vi "Clear Array.vi"(8 "error in (no error)":errorcluster, 11 "2DArrayManager in":refnum<class "2DArrayManager.lvclass">) -> (0 "error out":errorcluster, 3 "2DArrayManager out":refnum<class "2DArrayManager.lvclass">)   [LabVIEW 2020, in "OOPanel.lvlib" / "2DArrayManager.lvclass"]
doc: "Removes all panels from the layout but does NOT clean them up. They are marked as orphans so they can easily be reinserted as needed. Once orphaned, if the manager is cleaned up, the orphaned panels will be too."
uses:
  2DArrayManager.lvclass
  2DArrayManager.lvclass/2DArrayManager.ctl
  ArrayPanel/ArrayPanel.lvclass
  Panel/Panel.lvclass
  Manager/Manager.lvclass
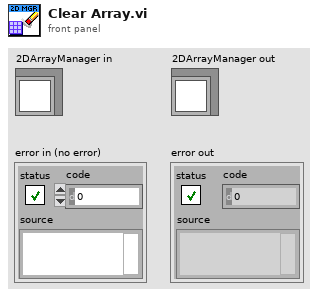
[diagram p1: front panel]
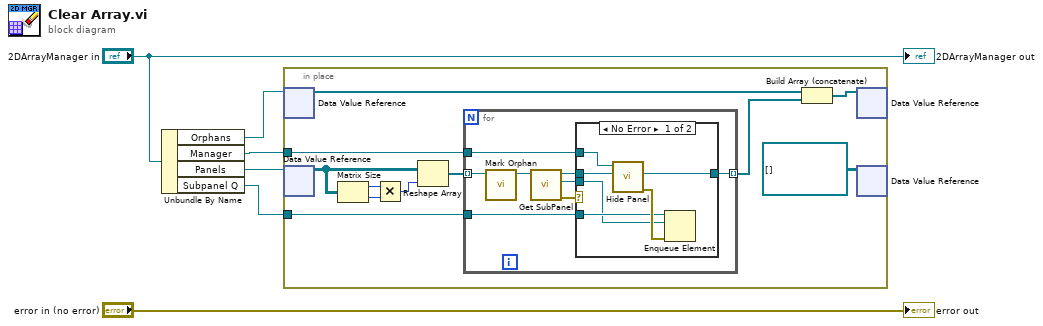
[diagram p0: block diagram]
diagram:
  n1 = Unbundle By Name("2DArrayManager in") -> ("Orphans"=w2:refnum<data-value>, "Manager"=w1:refnum<class "Manager.lvclass">, "Panels"=w4:refnum<data-value>, "Subpanel Q"=w3:refnum<queue>)
  n2 = in-place {
    in-place-border: w3 -> [w9]
    in-place-border: w1 -> [w8]
    n3 = in-place-dvr #1(w2) -> (w11:refnum<class "ArrayPanel.lvclass">[])  [unwired: 1 out]
    n4 = in-place-dvr #2(w4) -> (w17:refnum<class "ArrayPanel.lvclass">[][])  [unwired: 1 out]
    n5 = Matrix Size(0:w17) -> (1:w16:i32, 2:w15:i32)
    n6 = Multiply(x=w16, y=w15) -> (x*y=w14:i32)
    n7 = Reshape Array(w17, w14) -> (w12:refnum<class "ArrayPanel.lvclass">[])
    n8 = for {
      tunnel: w12 -> [w25] mode=indexing
      tunnel: w9 -> [w20]
      tunnel: w8 -> [w19]
      tunnel: [w18] -> w7 mode=indexing
      n9 = call "Mark Orphan.vi"("ArrayPanel in"=w25) -> ("ArrayPanel out"=w24:refnum<class "ArrayPanel.lvclass">)  [unwired: 9 in, 1 out]
      n10 = call "Get SubPanel.vi"("Panel in"=w24) -> ("error out"=w21:errorcluster, "SubPanel"=w22:refnum<vi>, "Panel out"=w23:refnum<class "ArrayPanel.lvclass">)  [unwired: 8 in]
      n11 = case shown="No Error" w21 {
        tunnel: w23 -> [w28 w32]
        tunnel: w22 -> [w27 _]
        tunnel: w20 -> [w30 _]
        tunnel: w19 -> [w29 _]
        tunnel: [w26 w32] -> w18
        frame No Error {
          n12 = call "Hide Panel.vi"("Panel In"=w28, "Manager in"=w29) -> ("error out"=w31:errorcluster, "Panel"=w26:refnum<class "ArrayPanel.lvclass">)  [unwired: 7 in, 1 out]
          n13 = Enqueue Element(queue=w30, element=w27, error in (no error)=w31) -> ()  [unwired: 1 in, 3 out]
        }
        frame Error {
        }
      }
    }
    n14 = Build Array (concatenate)(w11, w7) -> (w10:refnum<class "ArrayPanel.lvclass">[])
    n15 = in-place-dvr #1(w10) -> ()  [unwired: 2 out]
    n16 = in-place-dvr #2(refnum<class "ArrayPanel.lvclass">[][] [] ("data value")) -> ()  [unwired: 2 out]
  }
  "error out" <- "error in (no error)"
  "2DArrayManager out" <- "2DArrayManager in"
